vi "32xx_Decod_ON_OFF.vi"(11 "Réponse":string) -> (3 "ON/OFF":T1)   [LabVIEW 2020]
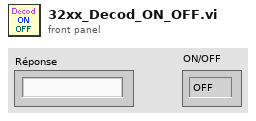
[diagram p1: front panel]
types:
  T1 = typedef "32xx_Enum_ON_OFF.ctl" = enum16{"OFF", "ON"}
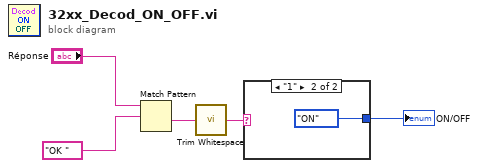
[diagram p0: block diagram]
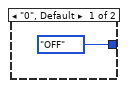
[diagram p2: hidden frame]
diagram:
  n1 = Match Pattern(string="Réponse", regular expression="OK " ("expression régulière")) -> (after substring=w5:string)  [unwired: 1 in, 3 out]
  n2 = call <vilib>:"Trim Whitespace.vi"("string"=w5) -> ("trimmed string"=w4:string)  [unwired: 1 in]
  n3 = case shown="\"1\"" w4 {
    tunnel: [32xx_Enum_ON_OFF."OFF" ("ON/OFF") 32xx_Enum_ON_OFF."ON" ("ON/OFF")] -> w1
    frame "0", Default {
    }
    frame "1" {
    }
  }
  "ON/OFF" <- w1
